vi "Test Binary Footprint of Data Type Of Boolean In Raw Data.vi"   [LabVIEW 2024]
types:
  T1 = enum16{"open", "open or create", "create or replace", "create", "open (read-only)"}
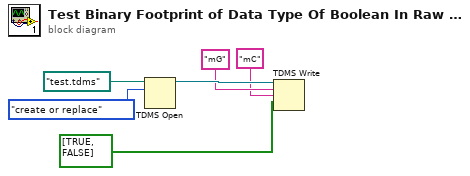
[diagram p0: block diagram]
diagram:
  n1 = TDMS Open(10:T1."create or replace" ("操作(0:open)"), 11:path "test.tdms" ("文件路径")) -> (3:w5:refnum<k34>)  [unwired: 5 in, 1 out]
  n2 = TDMS Write(0:w5, 5:"mG" ("组名称输入（无标题）"), 7:"mC" ("通道名输入（无标题）"), 9:bool[] [TRUE, FALSE]) -> ()  [unwired: 2 in, 4 out]
